vi "ErrorLoop.vi"(8 "Error In":errorcluster, 11 "Message Queues":T1) -> (0 "Error Out":errorcluster)   [LabVIEW 2017, in "Server.lvlib" / "ErrorLogger.lvlib"]
doc: "This Loop receives all errors and warnings coming from any other loop. It then validates if the error is critical, and if yes, it stops the Application by sending a UserEvent to the EHL.\nThis Loop also logs all Errors to a textfile."
uses:
  ErrorLogger.lvlib
  Message Queue/CommReferences.ctl
  Message Queue/MessageCluster.ctl
  ErrorLoopData.ctl
  TypeDefs/ServerINI.ctl
  Oracle/OracleData.ctl
  <vilib>/Utility/error.llb/Error Cluster From Error Code.vi
  <vilib>/ErrorRing/Error Ring.xnode
  Message Queue/Message Queue.lvlib
  Logging/Logging.lvlib
  Oracle/Oracle.lvlib
  Server.lvlib
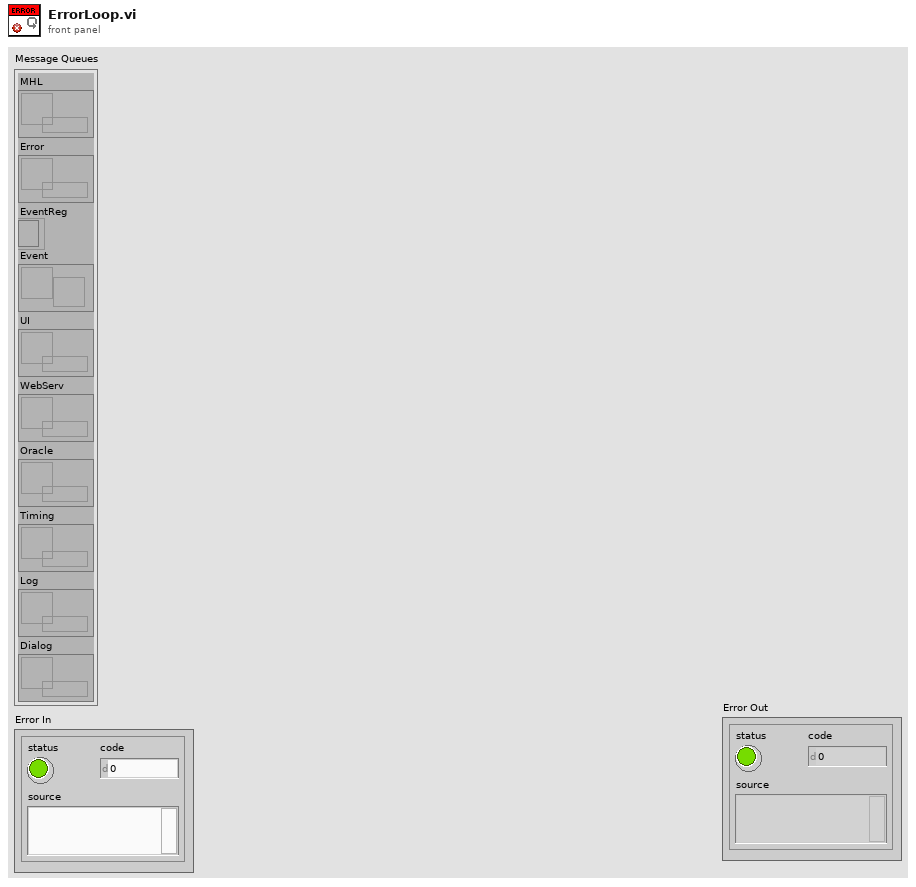
[diagram p1: front panel]
types:
  T1 = typedef "Server.lvlib/Message Queue.lvlib/CommReferences.ctl" = cluster{"MHL":refnum<queue>, "Error":refnum<queue>, "EventReg":refnum<event-registration>, "Event":refnum<user-event>, "UI":refnum<queue>, "WebServ":refnum<queue>, "Oracle":refnum<queue>, "Timing":refnum<queue>, "Log":refnum<queue>, "Dialog":refnum<queue>}
  T2 = typedef "Server.lvlib/ErrorLogger.lvlib/ErrorLoopData.ctl" = cluster{"CriticalErrors":i32[]}
  T3 = typedef "Server.lvlib/ServerINI.ctl" = cluster{"ClientTimeout (s)":u32, "LogPath":path, "CriticalErrors":i32[], "OracleData":T4}
  T4 = typedef "Server.lvlib/Oracle.lvlib/OracleData.ctl" = cluster{"DBname":string, "User":string, "Password":string}
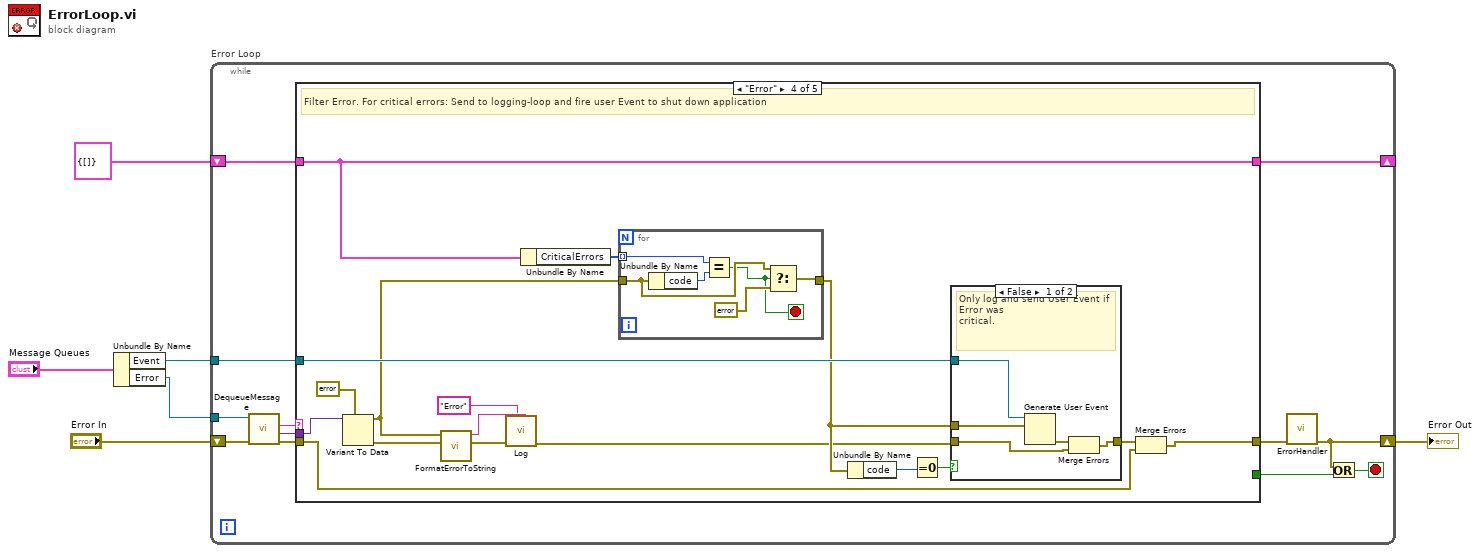
[diagram p0: block diagram]
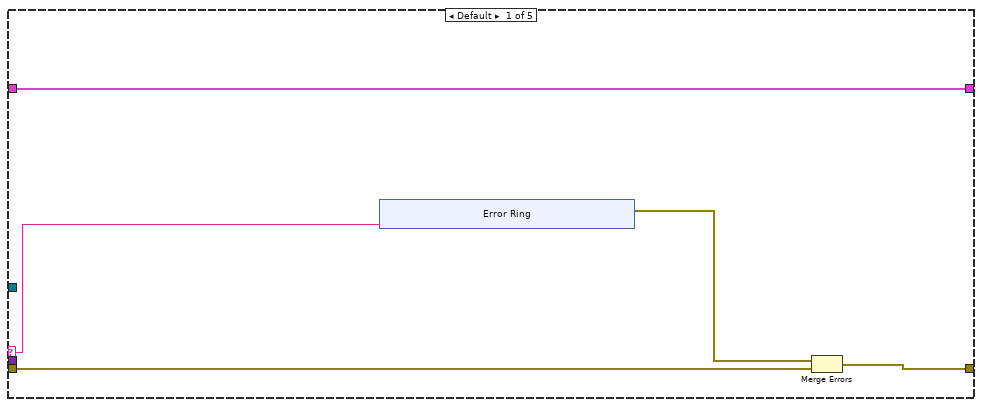
[diagram p2: hidden frame]
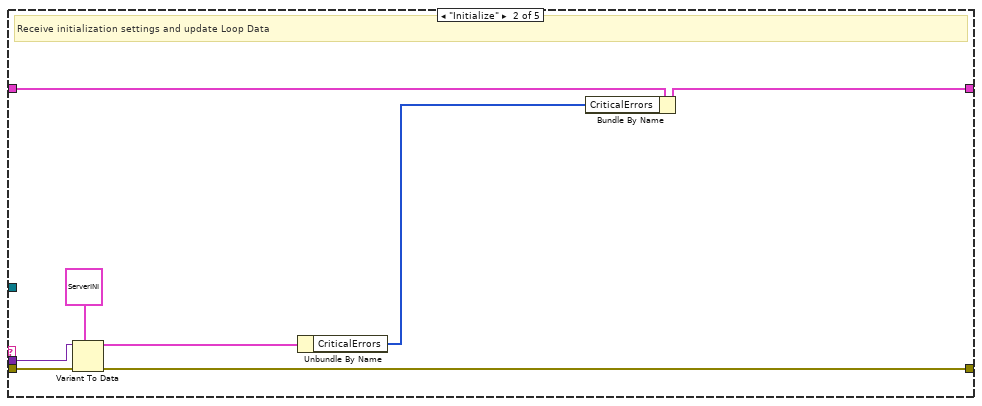
[diagram p3: hidden frame]
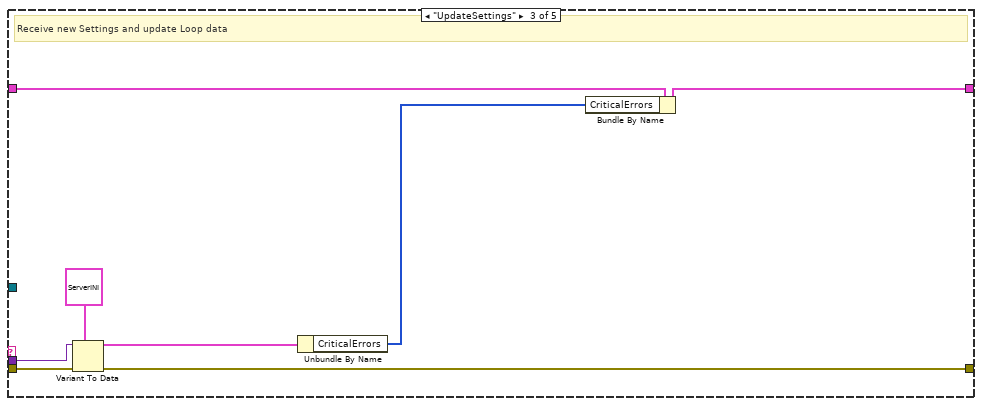
[diagram p4: hidden frame]
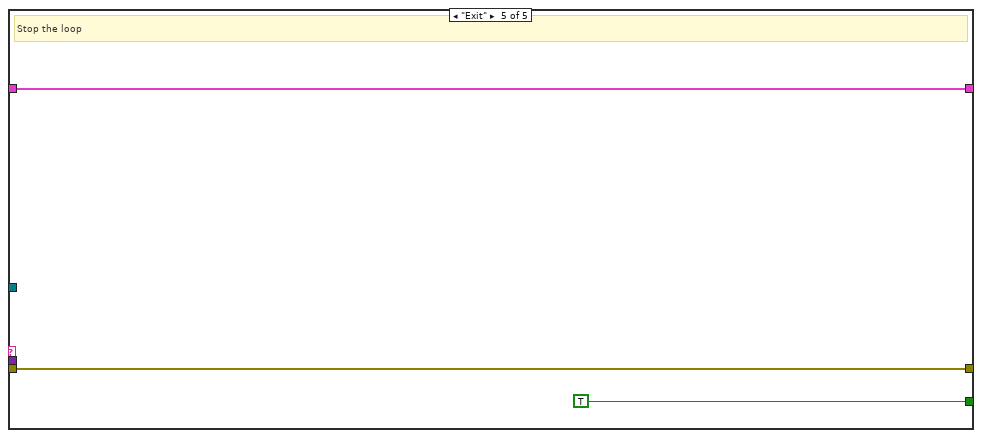
[diagram p6: hidden frame]
diagram:
  n1 = Unbundle By Name("Message Queues") -> ("Event"=w2:refnum<user-event>, "Error"=w3:refnum<queue>)
  n2 = while "Error Loop" {
    shift-right: [w7] -> w5
    shift-left: "Error In" -> [w18]
    tunnel: w3 -> [w16]
    tunnel: w2 -> [w11]
    shift-right: [w9] -> _
    shift-left: T2 {"CriticalErrors"=[]} ("ErrorLoopData") -> [w10]
    stop <- w8 stop-if-true
    n3 = call "DequeueMessage.vi"("error in (no error)"=w18, "Message Queue"=w16) -> ("error out"=w17:errorcluster, "Message Data"=w14:variant, "Message"=w15:string)  [unwired: 5 in, 2 out]
    n4 = case shown="\"Error\"" w15 {
      selector: w15 -> [w20 _ _ _ _]
      tunnel: [w22 w37 w45 w59 w78] -> w12
      tunnel: w17 -> [w23 w38 w46 w58 w78]
      tunnel: w14 -> [_ w36 w44 w61 _]
      tunnel: [_ _ _ _ TRUE] -> w13
      tunnel: w11 -> [_ _ _ w62 _]
      tunnel: w10 -> [w19 w34 w42 w54 w76]
      tunnel: [w19 w33 w41 w54 w76] -> w9
      frame Default {
        n5 = xnode "Error Ring"("parameter 0"=w20) -> ("error out"=w21:errorcluster)
        n6 = Merge Errors(w21, w23) -> (w22:errorcluster)
      }
      frame "Initialize" {
        # "Receive initialization settings and update Loop Data"
        n7 = Variant To Data(error in=w38, type=T3 {"ClientTimeout (s)"=30, "LogPath"=path "C:/Users/jgoebel/Documents/GitHub/AEDashboard/ServerLib/Data/ServerLog.tdms", "CriticalErrors"=[], "OracleData"={"DBname"="", "User"="", "Password"=""}} ("ServerINI"), Variant=w36) -> (data=w32:T3, error out=w37:errorcluster)
        n8 = Unbundle By Name(w32) -> ("CriticalErrors"=w31:i32[])
        n9 = Bundle By Name(cluster=w34, "CriticalErrors"=w31) -> (w33:T2)
      }
      frame "UpdateSettings" {
        # "Receive new Settings and update Loop data"
        n10 = Variant To Data(error in=w46, type=T3 {"ClientTimeout (s)"=30, "LogPath"=path "C:/Users/jgoebel/Documents/GitHub/AEDashboard/ServerLib/Data/ServerLog.tdms", "CriticalErrors"=[], "OracleData"={"DBname"="", "User"="", "Password"=""}} ("ServerINI"), Variant=w44) -> (data=w40:T3, error out=w45:errorcluster)
        n11 = Unbundle By Name(w40) -> ("CriticalErrors"=w39:i32[])
        n12 = Bundle By Name(cluster=w42, "CriticalErrors"=w39) -> (w41:T2)
      }
      frame "Error" {
        # "Filter Error. For critical errors: Send to logging-loop and fire user Event to shut down application"
        n13 = Variant To Data(type=errorcluster {"status"=FALSE, "code"=0, "source"=""} ("error constant"), Variant=w61) -> (data=w47:errorcluster, error out=w49:errorcluster)  [unwired: 1 in]
        n14 = call "FormatErrorToString.vi"("error in"=w49, "ErrorToLog"=w47) -> ("error out"=w52:errorcluster, "ErrorString"=w51:string)  [unwired: 8 in]
        n15 = call "Log.vi"("LogMessage"=w51, "Type"="Error", "Error In"=w52) -> ("Error Out"=w48:errorcluster)  [unwired: 8 in]
        n16 = Unbundle By Name(w54) -> ("CriticalErrors"=w53:i32[])
        n17 = for {
          tunnel: w53 -> [w75] mode=indexing
          tunnel: w47 -> [w73]
          tunnel: [w71] -> w57
          stop <- w70 stop-if-true
          n18 = Unbundle By Name(w73) -> ("code"=w74:i32)
          n19 = Equal?(x=w75, y=w74) -> (x = y?=w70:bool)
          n20 = Select(t=w73, s=w70, f=errorcluster {"status"=FALSE, "code"=0, "source"=""}) -> (s? t:f=w71:errorcluster)
        }
        n21 = Unbundle By Name(w57) -> ("code"=w56:i32)
        n22 = Equal To 0?(x=w56) -> (x = 0?=w55:bool)
        n23 = case shown="False" w55 {
          tunnel: [w66 w69] -> w63
          tunnel: w62 -> [w68 _]
          tunnel: w48 -> [w65 w69]
          tunnel: w57 -> [w64 _]
          frame False {
            # "Only log and send User Event if Error was\ncritical."
            n24 = Generate User Event(user event=w68, event data cluster=w64) -> (error out=w67:errorcluster)  [unwired: 2 in, 1 out]
            n25 = Merge Errors(w67, w65) -> (w66:errorcluster)
          }
          frame True {
            # "Error was filtered -> do nothing"
          }
        }
        n26 = Merge Errors(w63, w58) -> (w59:errorcluster)
      }
      frame "Exit" {
        # "Stop the loop"
      }
    }
    n27 = call "ErrorHandler.vi"("error in (no error)"=w12) -> ("error out"=w7:errorcluster)  [unwired: 10 in]
    n28 = Or(x=w7, y=w13) -> (x .or. y?=w8:bool)
  }
  "Error Out" <- w5
